vi "Get Attribute VAR.vi"(8 "error in":errorcluster, 10 "Attribute":string, 11 "ConfigFromJSON in":refnum<class "Config from JSON.lvclass">) -> (0 "error out":errorcluster, 2 "Value":variant, 3 "ConfigFromJSON out":refnum<class "Config from JSON.lvclass">)   [LabVIEW 2024, in "Config from JSON.lvclass"]
uses:
  Config from JSON.lvclass
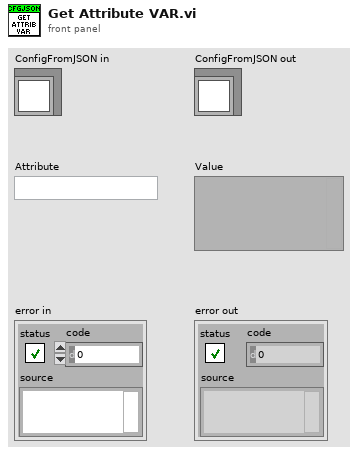
[diagram p1: front panel]
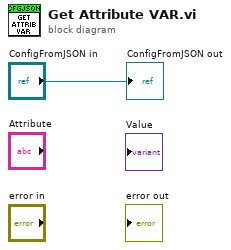
[diagram p0: block diagram]
diagram:
  "ConfigFromJSON out" <- "ConfigFromJSON in"
